vi "GetConstantConstructor.vi"(6 "error in":errorcluster, 9 "Constant in":refnum<class "Constant.lvclass">) -> (0 "error out":errorcluster, 3 "Constant out":refnum<class "Constant.lvclass">, 4 "constant":string)   [LabVIEW 2014, in "Raspberry Pi Compatible Compiler for LabVIEW.lvlib" / "Constant.lvclass"]
uses:
  Constant.lvclass
  Python/Parsing/Python Functions.lvlib
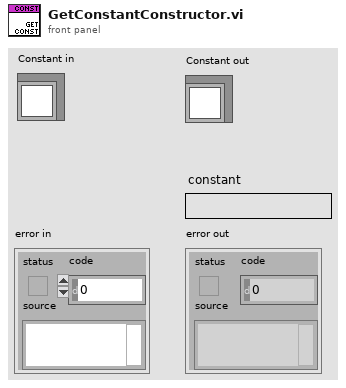
[diagram p1: front panel]
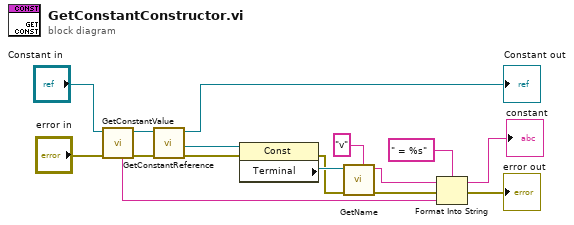
[diagram p0: block diagram]
diagram:
  n1 = call "GetConstantValue.vi"("error in"="error in", "Constant in"="Constant in") -> ("error out"=w5:errorcluster, "Constant out"=w4:refnum<class "Constant.lvclass">, "value"=w11:string)  [unwired: 5 in]
  n2 = call "GetConstantReference.vi"("error in"=w5, "Constant in"=w4) -> ("error out"=w3:errorcluster, "reference out"=w2:refnum<vi>, "Constant out"=→"Constant out":refnum<class "Constant.lvclass">)  [unwired: 5 in]
  n3 = property class="Const"(reference=w2, error in=w3) -> (error out=w6:errorcluster, "Terminal"=w7:refnum<vi>)  [unwired: 1 out]
  n4 = call "GetName.vi"("base name"="v", "error in"=w6, "GObj Refnum"=w7) -> ("error out"=w13:errorcluster, "name"=w12:string)  [unwired: 6 in, 1 out]
  n5 = Format Into String(format string=" = %s", initial string=w12, error in=w13, w11) -> (resulting string=→"constant":string, error out=→"error out":errorcluster)
